vi "SaveSystemConfigurationUI.vi"(8 "error in (no error)":errorcluster, 11 "SoftwareSetup in":refnum<class "SoftwareSetup.lvclass">) -> (0 "error out":errorcluster, 3 "SoftwareSetup out":refnum<class "SoftwareSetup.lvclass">)   [LabVIEW 2019, in "SoftwareSetup.lvlib" / "SoftwareSetup.lvclass"]
uses:
  SoftwareSetup.lvclass
  C:/Program Files (x86)/National Instruments/LabVIEW 2019/vi.lib/NI/Event Source Actor/Event Source/Event Source/Event Source.lvclass
  SoftwareSetup.lvclass/SoftwareSetup.ctl
  SystemSetup/SystemSetup/SystemConfiguration.lvclass
  C:/Program Files (x86)/National Instruments/LabVIEW 2019/vi.lib/NI/Event Source Actor/Event Source/Event/Event.lvclass
  <vilib>/NI/Event Source Actor/Event Source/Event/Event.lvclass/Event.ctl
  SystemSetup/SystemSetup/SystemSetup.lvclass
  <vilib>/NI/Event Source Actor/Event Source/Event/Event.lvclass
  <vilib>/NI/Event Source Actor/Event Source/Event Source/Event Source.lvclass
  <vilib>/Utility/config.llb/NI_LVConfig.lvlib
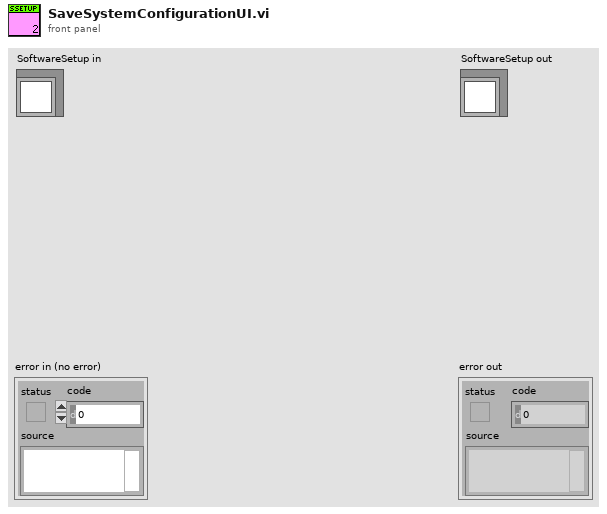
[diagram p1: front panel]
types:
  T1 = typedef "SoftwareSetup.lvlib/DataBase.ctl" = cluster{"Connection String Expression":string, "User ID":string, "Password":string}
  T2 = typedef "SoftwareSetup.lvlib/Local Report.ctl" = cluster{"Report Path":path, "Report  Format":enum16{"CSV", "XML", "PDF", "Excel", "TXT"}, "Disabled State":bool, "Customer name":string}
  T3 = typedef "SoftwareSetup.lvlib/Localization.ctl" = cluster{"Language":enum16{"English", "Chinese"}}
  T4 = typedef "SoftwareSetup.lvlib/Preferences.ctl" = cluster{"Station ID":string, "IP Address":string, "Password":string}
  T5 = typedef "SoftwareSetup.lvlib/User Manager.ctl" = cluster{"Current User Manager File":string, "Login on start":bool}
  T6 = typedef "SoftwareSetup.lvlib/Multiple UUT Settings.ctl" = cluster{"Number of Tests Sockets":u8, "Synchronization":enum16{"Don't Synchronize", "Serial", "Parallel", "One Thread Only"}}
  T7 = typedef "SoftwareSetup.lvlib/Sequence.ctl" = cluster{"Sequence Folder Path":path}
  T8 = cluster{"DataBase":T1, "Local Report":T2, "Localization":T3, "Preferences":T4, "User Manager":T5, "Multiple UUT Settings":T6, "Sequence":T7}
  T9 = typedef "Multiple UUT Settings.ctl" = cluster{"Number of Tests Sockets":u8, "Synchronization":enum16{"Don't Synchronize", "Serial", "Parallel", "One Thread Only"}}
  T10 = typedef "Sequence.ctl" = cluster{"Sequence Folder Path":path}
  T11 = typedef "NI_LVConfig.lvlib/Config Data RefNum.ctl" = refnum<k1>
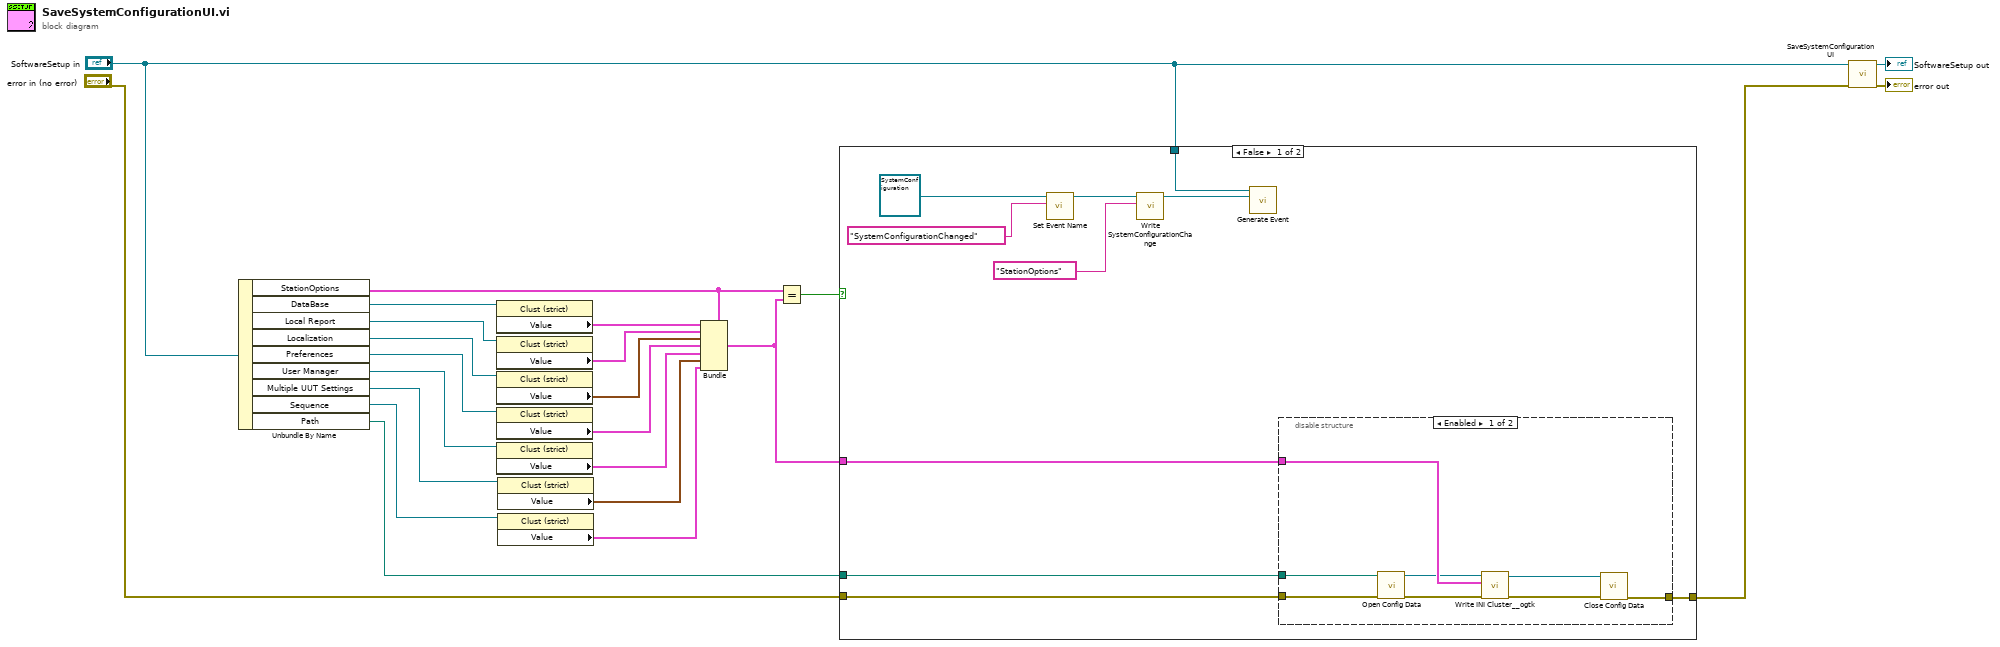
[diagram p0: block diagram]
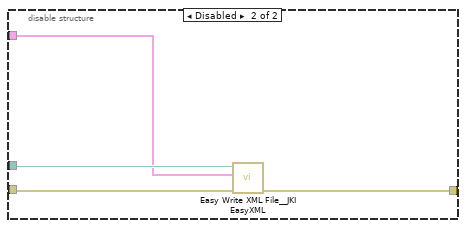
[diagram p2: hidden frame]
diagram:
  n1 = Unbundle By Name("SoftwareSetup in") -> ("StationOptions"=w6:T8, "DataBase"=w21:refnum<vi>, "Local Report"=w17:refnum<vi>, "Localization"=w16:refnum<vi>, "Preferences"=w15:refnum<vi>, "User Manager"=w14:refnum<vi>, "Multiple UUT Settings"=w5:refnum<vi>, "Sequence"=w2:refnum<vi>, "Path"=w3:path)
  n2 = property class="Clust (strict)"(reference=w21) -> ("Value"=w13:T1)  [unwired: 1 in, 2 out]
  n3 = property class="Clust (strict)"(reference=w17) -> ("Value"=w12:T2)  [unwired: 1 in, 2 out]
  n4 = property class="Clust (strict)"(reference=w16) -> ("Value"=w11:T3)  [unwired: 1 in, 2 out]
  n5 = property class="Clust (strict)"(reference=w15) -> ("Value"=w10:T4)  [unwired: 1 in, 2 out]
  n6 = property class="Clust (strict)"(reference=w14) -> ("Value"=w9:T5)  [unwired: 1 in, 2 out]
  n7 = property class="Clust (strict)"(reference=w5) -> ("Value"=w4:T9)  [unwired: 1 in, 2 out]
  n8 = property class="Clust (strict)"(reference=w2) -> ("Value"=w1:T10)  [unwired: 1 in, 2 out]
  n9 = Bundle(cluster=w6, "DataBase"=w13, "Local Report"=w12, "Localization"=w11, "Preferences"=w10, "User Manager"=w9, "Multiple UUT Settings"=w4, "Sequence"=w1) -> (w8:T8)
  n10 = Equal?(x=w6, y=w8) -> (x = y?=w20:bool)
  n11 = case shown="False" w20 {
    tunnel: "error in (no error)" -> [w33 w46]
    tunnel: [w32 w46] -> w7
    tunnel: w3 -> [w31 _]
    tunnel: w8 -> [w30 _]
    tunnel: "SoftwareSetup in" -> [w25 _]
    frame False {
      n12 = call <vilib>:"Set Event Name.vi"("Name (Generic)"="SystemConfigurationChanged", "Event In"=refnum<class "SystemConfiguration.lvclass"> refnum ("SystemSetup.lvlib:SystemConfiguration.lvclass")) -> ("Event Out"=w27:refnum<class "SystemConfiguration.lvclass">)  [unwired: 9 in]
      n13 = call-dynamic "Write SystemConfigurationChange.vi"("SystemConfigurationChange"="StationOptions", "SystemConfiguration in"=w27) -> ("SystemConfiguration out"=w26:refnum<class "SystemConfiguration.lvclass">)  [unwired: 8 in, 1 out]
      n14 = call <vilib>:"Generate Event.vi"("Event"=w26, "Event Source In"=w25) -> ()  [unwired: 8 in, 2 out]
      n15 = disable-structure shown="Enabled" {
        disable-tunnel: w33 -> [w41 w44]
        disable-tunnel: [w40 w42] -> w32
        disable-tunnel: w31 -> [w39 w45]
        disable-tunnel: w30 -> [w38 w43]
        frame Enabled {
          n16 = call <vilib>:"Open Config Data.vi"("error in (no error)"=w41, "configuration file path"=w39) -> ("error out"=w36:errorcluster, "refnum"=w37:T11)  [unwired: 7 in, 1 out]
          n17 = call <userlib>:"Write INI Cluster__ogtk.vi"("error in (no error)"=w36, "INI Fomatted Cluster"=w38, "refnum"=w37) -> ("error out"=w34:errorcluster, "dup refnum"=w35:T11)  [unwired: 7 in]
          n18 = call <vilib>:"Close Config Data.vi"("error in (no error)"=w34, "refnum"=w35) -> ("error out"=w40:errorcluster)  [unwired: 8 in, 1 out]
        }
        frame Disabled {
          n19 = call <vilib>:"Easy Write XML File__JKI EasyXML.vi"("error in (no error)"=w44, "LabVIEW Data"=w43, "XML File Path"=w45) -> ("error out"=w42:errorcluster)  [unwired: 7 in, 1 out]
        }
      }
    }
    frame True {
    }
  }
  n20 = call-parent "SaveSystemConfigurationUI.vi"("error in (no error)"=w7, "SystemSetup in"="SoftwareSetup in") -> ("error out"=→"error out":errorcluster, "SystemSetup out"=→"SoftwareSetup out":refnum<class "SoftwareSetup.lvclass">)  [unwired: 8 in]
